vi "HW6p1_Task1_nguyejk.vi"() -> ()   [LabVIEW 2016]
panel:
  out "Last Day":dbl
  out "Days":dbl
  out "Actual Saving":dbl
  in  "Desired Saving":dbl
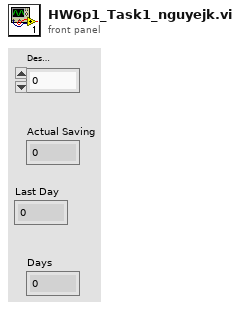
[diagram p1: front panel]
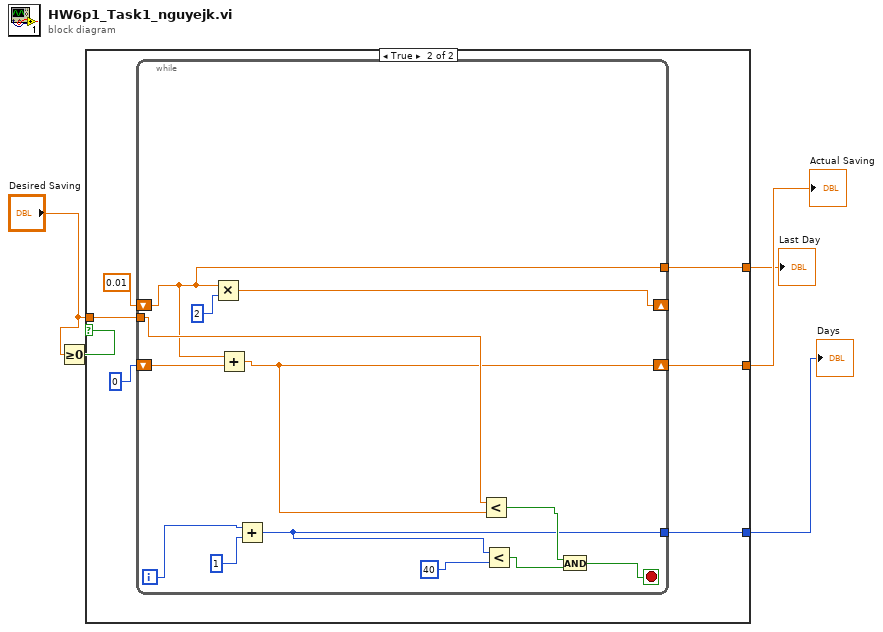
[diagram p0: block diagram]
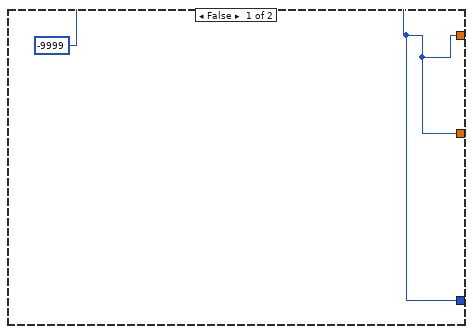
[diagram p2: hidden frame]
diagram:
  n1 = Greater Or Equal To 0?(x="Desired Saving") -> (x >= 0?=w5:bool)
  n2 = case shown="True" w5 {
    tunnel: [w6 w12] -> w4
    tunnel: "Desired Saving" -> [_ w11]
    tunnel: [w6 w8] -> w2
    tunnel: [w6 w7] -> w1
    frame False {
      w6 = -9999
    }
    frame True {
      n3 = while {
        shift-right: [w21] -> _
        shift-left: 0.01 -> [w18]
        tunnel: [w13] -> w12
        tunnel: w11 -> [w22]
        shift-right: [w19] -> w8
        shift-left: 0 -> [w20]
        tunnel: [w18] -> w7
        i -> [w24]
        stop <- w16 stop-if-true
        n4 = Multiply(x=w18, y=2) -> (x*y=w21:dbl)
        n5 = Add(x=w18, y=w20) -> (x+y=w19:dbl)
        n6 = Add(x=w24, y=1) -> (x+y=w13:i32)
        n7 = Less?(x=w22, y=w19) -> (x < y?=w17:bool)
        n8 = Less?(x=w13, y=40) -> (x < y?=w15:bool)
        n9 = And(x=w17, y=w15) -> (x .and. y?=w16:bool)
      }
    }
  }
  "Actual Saving" <- w2
  "Days" <- w4
  "Last Day" <- w1
